vi "GetAllFiles.vi"(3 "error in (no error)":errorcluster, 4 "Pattern":string, 5 "FolderPath":path) -> (0 "error out":errorcluster, 2 "Files":string[](array[string]))   [LabVIEW 2013]
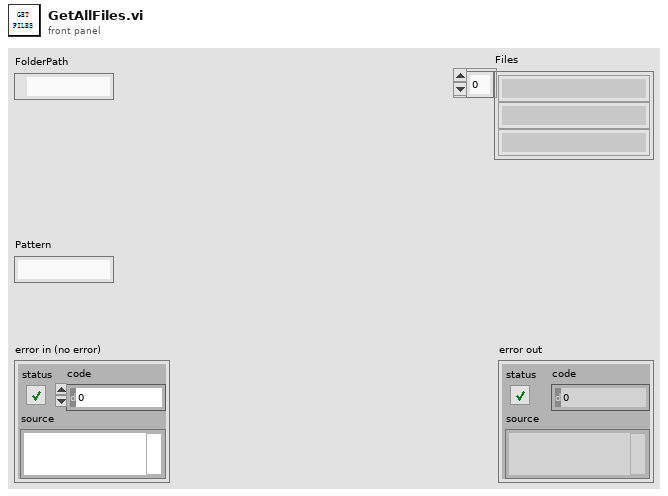
[diagram p1: front panel]
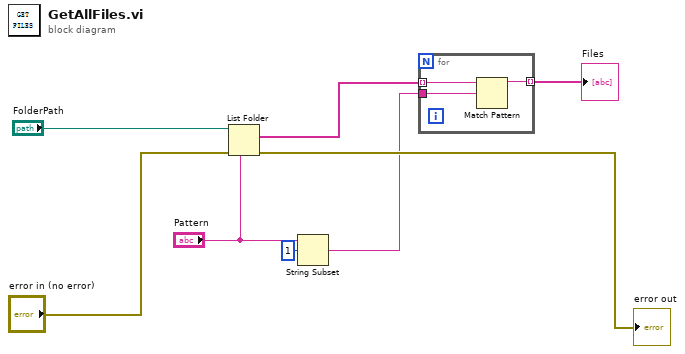
[diagram p0: block diagram]
diagram:
  n1 = List Folder(path="FolderPath", pattern="Pattern", error in="error in (no error)") -> (filenames=w1:string[], error out=→"error out":errorcluster)  [unwired: 1 in, 2 out]
  n2 = String Subset(string="Pattern", offset (0)=1) -> (substring=w2:string)  [unwired: 1 in]
  n3 = for {
    tunnel: w1 -> [w11] mode=indexing
    tunnel: [w10] -> w5 mode=indexing
    tunnel: w2 -> [w9]
    n4 = Match Pattern(string=w11, regular expression=w9) -> (before substring=w10:string)  [unwired: 1 in, 3 out]
  }
  "Files" <- w5
